vi "Set Units.vi"(8 "error in (no error)":errorcluster caption="错误输入（无错误）", 10 "Units":string, 11 "Channel输入":refnum<class "Channel.lvclass">) -> (0 "error out":errorcluster caption="错误输出", 3 "Channel输出":refnum<class "Channel.lvclass">)   [LabVIEW 2013, in "Hierarchy Framework.lvlib" / "Channel.lvclass"]
uses:
  Channel.lvclass
  Channel.lvclass/Channel.ctl
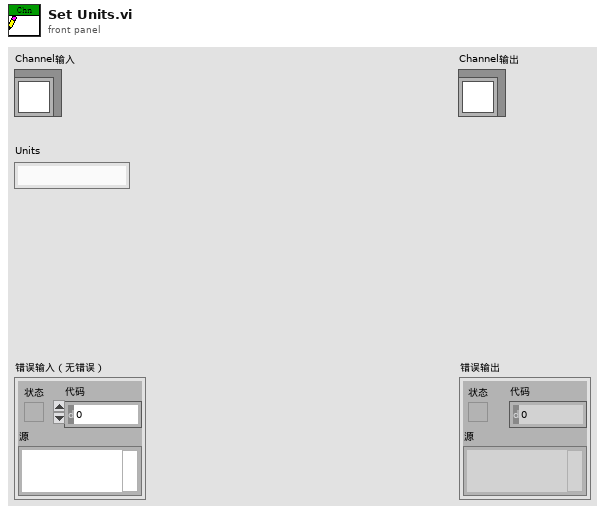
[diagram p1: front panel]
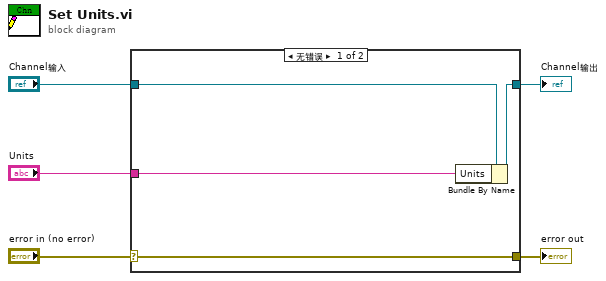
[diagram p0: block diagram]
diagram:
  n1 = case shown="无错误" "error in (no error)" {
    selector: "error in (no error)" -> [w9 w10]
    tunnel: [w9 w10] -> w4
    tunnel: [w7 w11] -> w2
    tunnel: "Channel输入" -> [w8 w11]
    tunnel: "Units" -> [w6 _]
    frame No Error {
      n2 = Bundle By Name(cluster=w8, "Units"=w6) -> (w7:refnum<class "Channel.lvclass">)
    }
    frame Error {
    }
  }
  "error out" <- w4
  "Channel输出" <- w2
